vi "Log Event.vi"(8 "error in (no error)":errorcluster, 10 "Event Text":string, 11 "MWWL Verification in":refnum<class "MWWL Verification.lvclass">) -> (0 "error out":errorcluster, 3 "MWWL Verification out":refnum<class "MWWL Verification.lvclass">)   [LabVIEW 2018, in "MWWL Verification.lvlib" / "MWWL Verification.lvclass"]
uses:
  MWWL Verification.lvclass
  MWWL Verification.lvclass/MWWL Verification.ctl
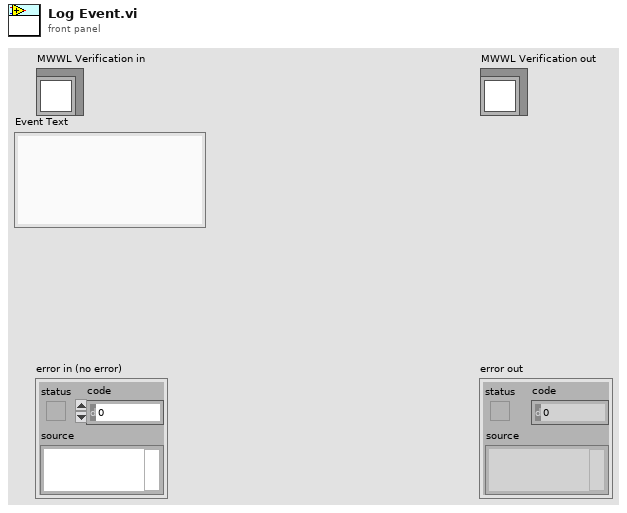
[diagram p1: front panel]
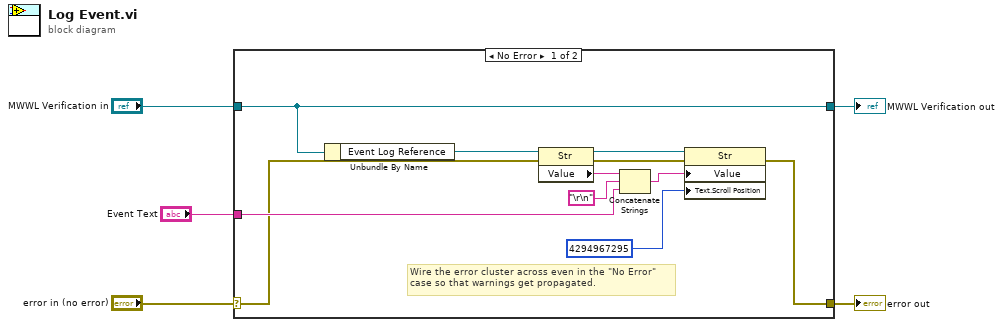
[diagram p0: block diagram]
diagram:
  n1 = case shown="No Error" "error in (no error)" {
    selector: "error in (no error)" -> [w7 w18]
    tunnel: [w6 w18] -> w4
    tunnel: [w8 w17] -> w2
    tunnel: "MWWL Verification in" -> [w8 w17]
    tunnel: "Event Text" -> [w9 _]
    frame No Error {
      # "Wire the error cluster across even in the \"No Error\"\ncase so that warnings get propagated."
      n2 = Unbundle By Name(w8) -> ("Event Log Reference"=w10:refnum<vi>)
      n3 = property class="Str"(reference=w10, error in=w7) -> (reference out=w13:refnum<vi>, error out=w14:errorcluster, "Value"=w11:string)
      n4 = Concatenate Strings(w11, "\r\n", w9) -> (w15:string)
      n5 = property class="Str"(reference=w13, error in=w14, "Value"=w15, "Text.Scroll Position"=u32 4294967295) -> (error out=w6:errorcluster)  [unwired: 1 out]
    }
    frame Error {
    }
  }
  "error out" <- w4
  "MWWL Verification out" <- w2
